vi "LV Exp2.vi"() -> ()   [LabVIEW 2009]
uses:
  <vilib>/NXT/Block Support/NXT_InputPort.ctl
  <vilib>/NXT/Dual Mode Library/Waits/Wait_Num(msec).vi
  <vilib>/NXT/Dual Mode Library/Display/drawText.vi
panel:
  out "Analog Value":i16
  in  "stop":bool
  # "HiTechnic Experimenter's Kit\n\n                        Experiment 2 -Six LEDs and Pot.\nThis program reads the status of the potentiometer on port A0 and\noutput the value read to the LEDs connected to B0 - B5.\n\nSee Experimenter's Kit Handbook for the SuperPro for\nmore information or go to www.hitechnic.com.\n\n(c) HiTechnic 2011"
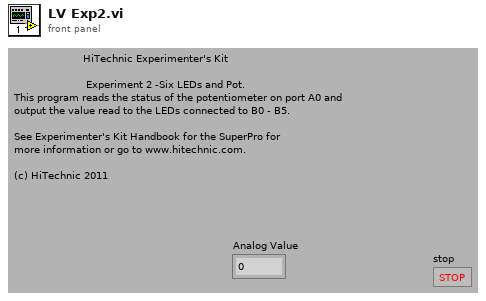
[diagram p1: front panel]
types:
  T1 = typedef "NXT_InputPort.ctl" = u8
  T2 = typedef "LVHSConnector.ctl" = cluster{"error":errorcluster, "address":string, "NXT #":i32, "Show Error":bool, "Connection":u16}
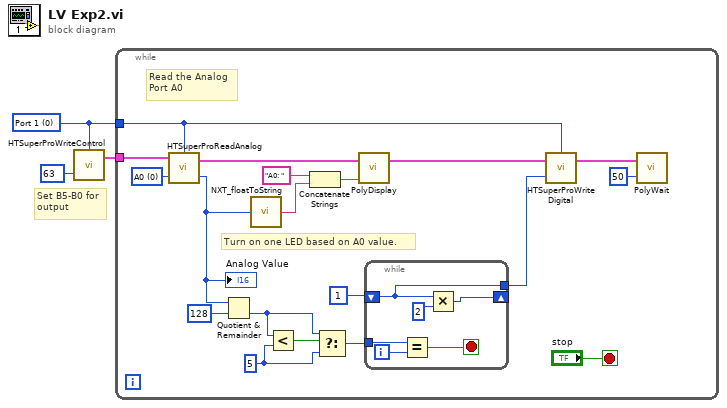
[diagram p0: block diagram]
diagram:
  w1 = T1 0 items=["Port 1", "Port 2", "Port 3", "Port 4"] ("Port")
  # "Set B5-B0 for\noutput"
  n1 = call "HTSuperProWriteControl.vi"("Digital Value"=u8 63, "Port"=w1) -> ("NXT"=w3:T2)  [unwired: 3 in]
  n2 = while {
    tunnel: w1 -> [w21]
    tunnel: w3 -> [w22]
    stop <- "stop" stop-if-true
    w13 = i16 5 ("y")
    w19 = u8 0 items=["A0", "A1", "A2", "A3"] ("Analog Port")
    # "Turn on one LED based on A0 value."
    # "Read the Analog\nPort A0"
    n3 = call "HTSuperProReadAnalog.vi"("Analog Port"=w19, "NXT"=w22, "Port"=w21) -> ("Analog Value"=w7:i16, "NXT"=w11:T2)  [unwired: 1 in]
    "Analog Value" <- w7
    n4 = Quotient & Remainder(x=w7, y=i16 128) -> (floor(x/y)=w14:i16)  [unwired: 1 out]
    n5 = call <vilib>:"NXT_floatToString.vi"("number"=w7) -> ("string"=w8:string)
    n6 = Less?(x=w14, y=w13) -> (x < y?=w15:bool)
    n7 = Concatenate Strings("A0: " ("string"), w8) -> (w10:string)
    n8 = Select(t=w14, s=w15, f=w13) -> (s? t:f=w12:i16)
    n9 = call-poly <vilib>:"PolyDisplay.vi"("Text"=w10, "NXT"=w11) -> ("NXT"=w6:T2)  [unwired: 2 in]
    n10 = while {
      tunnel: w12 -> [w27]
      shift-right: [w24] -> _
      shift-left: u8 1 ("Digital Value") -> [w23]
      tunnel: [w23] -> w16
      i -> [w28]
      stop <- w26 stop-if-true
      n11 = Equal?(x=w27, y=w28) -> (x = y?=w26:bool)
      n12 = Multiply(x=w23, y=u8 2) -> (x*y=w24:u8)
    }
    n13 = call "HTSuperProWriteDigital.vi"("Digital Value"=w16, "NXT"=w6, "Port"=w21) -> ("NXT"=w5:T2)  [unwired: 2 in]
    n14 = call-poly <vilib>:"PolyWait.vi"("Time (100 msec)"=u32 50, "NXT"=w5) -> ()  [unwired: 2 in, 1 out]
  }
